vi "Auto Number Retrieve Record.vi"(8 "error in (no error)":errorcluster, 11 "Statement Refnum":T1) -> (0 "error out":errorcluster, 2 "Auto Number Record":T2, 3 "Statement Refnum":T1)   [LabVIEW 2011]
uses:
  Auto Number Record.ctl
  SI.LIB/ODBC/SQL Controls/Statement Refnum.ctl
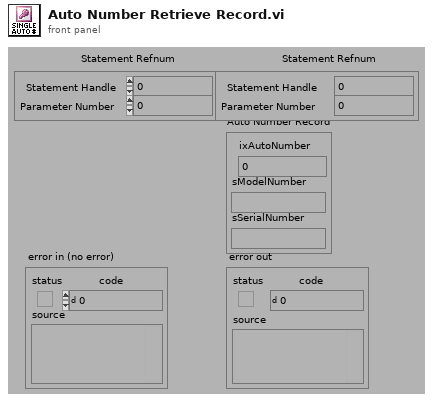
[diagram p1: front panel]
types:
  T1 = typedef "Statement Refnum.ctl" = cluster{"Statement Handle":i32, "Parameter Number":u16}
  T2 = typedef "Auto Number Record.ctl" = cluster{"ixAutoNumber":i32, "sModelNumber":string, "sSerialNumber":string}
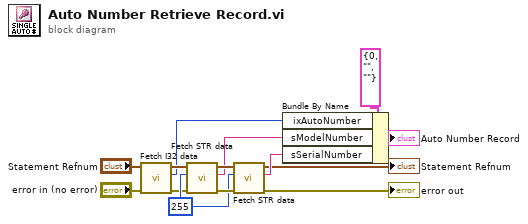
[diagram p0: block diagram]
diagram:
  w8 = 255 ("Buffer Size")
  n1 = call "Fetch I32 data.vi"("error in (no error)"="error in (no error)", "Statement Refnum"="Statement Refnum") -> ("error out"=w4:errorcluster, "Data"=w3:i32, "Statement Refnum"=w6:T1)  [unwired: 3 out]
  n2 = call "Fetch STR data.vi"("error in (no error)"=w4, "Buffer Size"=w8, "Statement Refnum"=w6) -> ("error out"=w14:errorcluster, "Data"=w10:string, "Statement Refnum"=w13:T1)  [unwired: 2 out]
  n3 = call "Fetch STR data.vi"("error in (no error)"=w14, "Buffer Size"=w8, "Statement Refnum"=w13) -> ("error out"=→"error out":errorcluster, "Data"=w9:string, "Statement Refnum"=→"Statement Refnum":T1)  [unwired: 2 out]
  n4 = Bundle By Name(cluster=T2 {"ixAutoNumber"=0, "sModelNumber"="", "sSerialNumber"=""} ("Field Data Information"), "ixAutoNumber"=w3, "sModelNumber"=w10, "sSerialNumber"=w9) -> (→"Auto Number Record":T2)
